vi "Record Fiducial.vi"(9 "CH index":i32, 10 "XYZ":dbl[](array[numeric]), 11 "input cluster":T1) -> (2 "All fiducials recorded":bool, 3 "output cluster":T1)   [LabVIEW 2021, in "Component Tray.lvclass"]
uses:
  Component Tray.lvclass
  Find Component.ctl
  Controller/Camera/Machine Vision.ctl
  Controller/Camera/Camera.lvclass
panel:
  out "XYZTheta":dbl[](array[numeric]) format="%.6g"
  out "CH1 XYZ":dbl[](array[numeric])
  out "Sensor ID Location":dbl[](array[numeric])
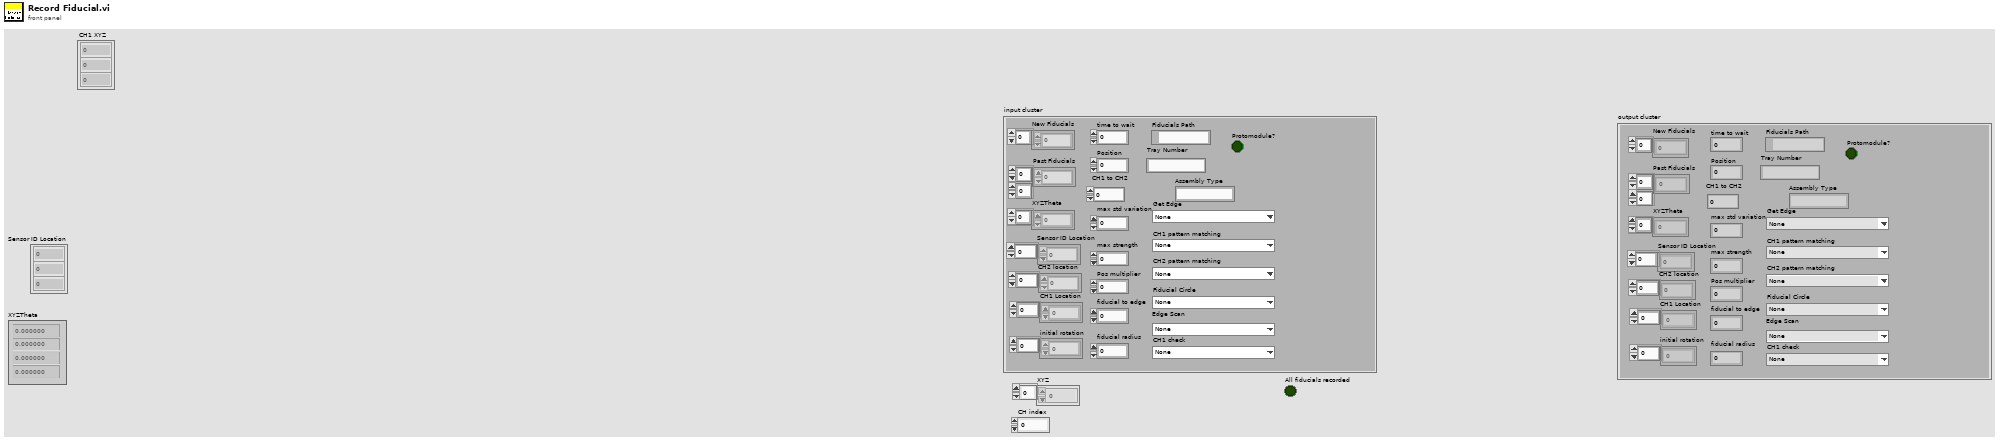
[diagram p1: front panel]
types:
  T1 = typedef "Component Tray.lvclass/Find Component.ctl" = cluster{"New Fiducials":dbl[], "Past Fiducials":dbl[][], "XYZTheta":dbl[], "Fiducials Path":path, "Position":i32, "CH1 Location":dbl[], "Sensor ID Location":dbl[], "initial rotation":dbl[], "CH2 location":dbl[], "max std variation":dbl, "max strength":dbl, "CH2 pattern matching":T2, "Fiducial Circle":T2, "Get Edge":T2, "Pos multiplier":dbl, "time to wait":u32, "fiducial to edge":dbl, "Protomodule?":bool, "Assembly Type":string, "CH1 to CH2":dbl, "Tray Number":string, "fiducial radius":dbl, "4 fiducials?":bool, "CH1 check":T2, "Edge Scan":T2, "CH1 pattern matching":T2, "Sensor Thickness":dbl}
  T2 = typedef "Camera.lvclass/Machine Vision.ctl" = enum16{"None", "Assembly Tray Circle", "Assembly Tray Fiducial", "Partial Hexaboard", "sensor edge init", "HB edge init", "sensor edge pos1", "sensor edge pos2", "HB edge pos1", "HB edge pos2", "Sensor CH1-2", "HB CH1", "HB CH2", "V3 Sensor Circle", "Hexaboard Circle", "sensor CH1 check", "HB CH1 check "}
  T3 = typedef "File Paths.ctl" = cluster{"Glue Pattern Folder":path, "Carrier Tray Folder":path, "Pick Up Tool Fixture Folder":path, "Components Folder":path, "Bellows Tool Offset.txt":path, "Pick Up Tool Offset.txt":path, "Dispense Tip Offset.txt":path, "Log Files":path, "Gantry Assembly Map.txt":path, "Syringe and offset map.txt":path, "Controllers Folder":path, "Local dbase config":path}
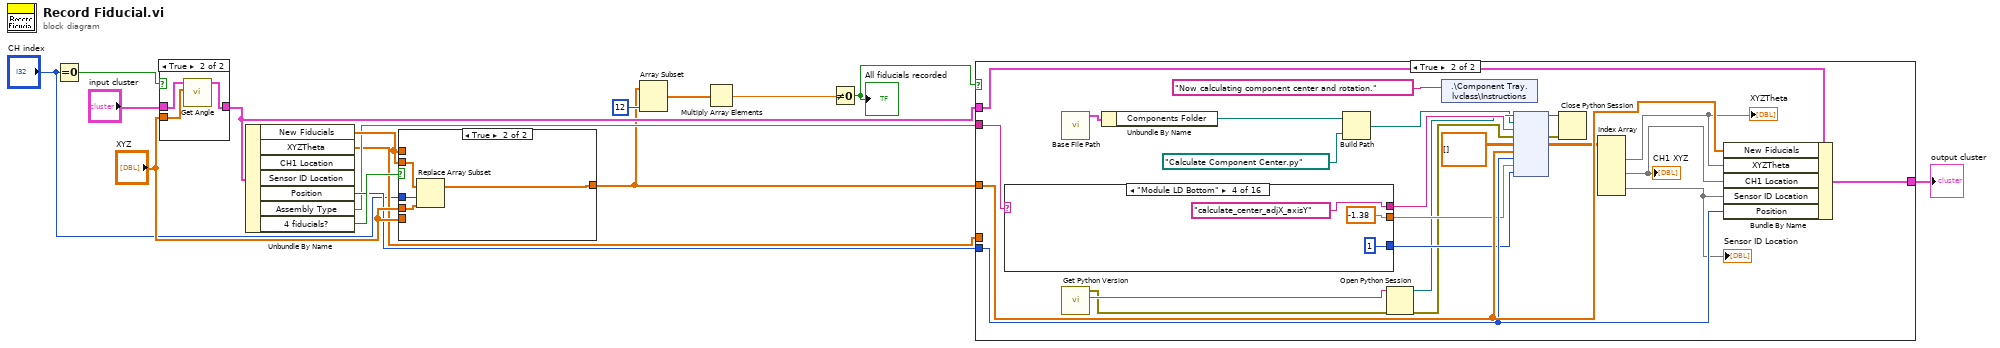
[diagram p0: block diagram]
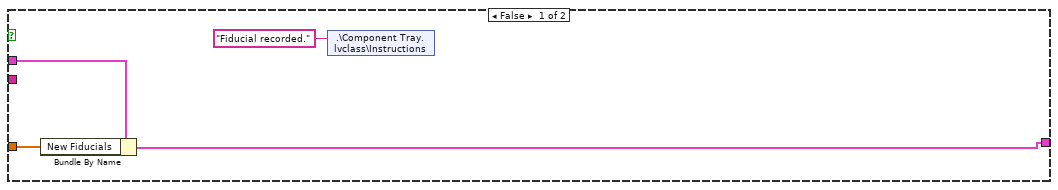
[diagram p2: hidden frame]
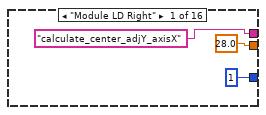
[diagram p3: hidden frame]
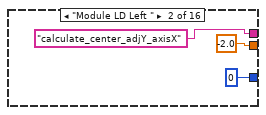
[diagram p4: hidden frame]
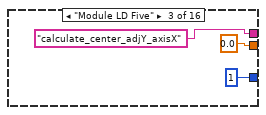
[diagram p5: hidden frame]
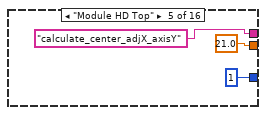
[diagram p6: hidden frame]
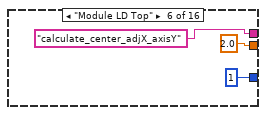
[diagram p7: hidden frame]
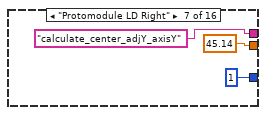
[diagram p8: hidden frame]
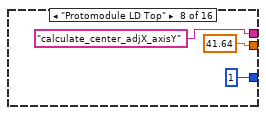
[diagram p9: hidden frame]
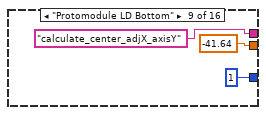
[diagram p10: hidden frame]
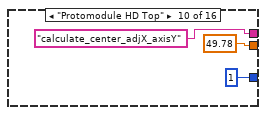
[diagram p11: hidden frame]
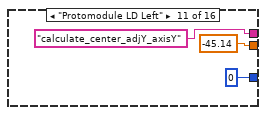
[diagram p12: hidden frame]
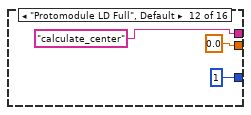
[diagram p13: hidden frame]
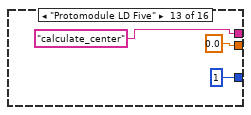
[diagram p14: hidden frame]
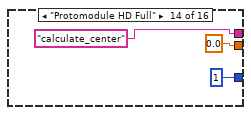
[diagram p15: hidden frame]
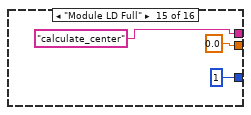
[diagram p16: hidden frame]
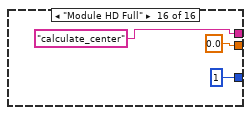
[diagram p17: hidden frame]
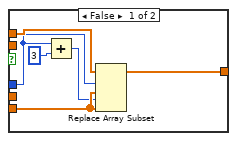
[diagram p19: hidden frame]
diagram:
  n1 = Equal To 0?(x="CH index") -> (x = 0?=w3:bool)
  n2 = case shown="True" w3 {
    tunnel: "input cluster" -> [w17 w20]
    tunnel: [w17 w19] -> w5
    tunnel: "XYZ" -> [_ w18]
    frame False {
    }
    frame True {
      n3 = call "Get Angle.vi"("array"=w18, "input cluster"=w20) -> ("output cluster"=w19:T1)  [unwired: 8 in, 1 out]
    }
  }
  n4 = Unbundle By Name(w5) -> ("New Fiducials"=w16:dbl[], "XYZTheta"=w6:dbl[], "Position"=w8:i32, "Assembly Type"=w7:string, "4 fiducials?"=w15:bool)  [unwired: 2 out]
  n5 = case shown="True" w15 {
    tunnel: w16 -> [w26 _]
    tunnel: "XYZ" -> [w25 _]
    tunnel: [w22 w27] -> w2
    tunnel: w16 -> [_ w30]
    tunnel: "XYZ" -> [_ w29]
    tunnel: "CH index" -> [w21 w28]
    frame False {
      n6 = Add(x=w21, y=3) -> (x+y=w23:i32)
      n7 = Replace Array Subset "Replace Array Subset"(array=w26, new element #1=w25, index #1=w21, new element #2=w25, index #2=w23) -> (w22:dbl[])
    }
    frame True {
      n8 = Replace Array Subset "Replace Array Subset"(array=w30, new element=w29, index=w28) -> (w27:dbl[])
    }
  }
  n9 = Array Subset "Array Subset"(array=w2, length=12) -> (w10:dbl[])  [unwired: 1 in]
  n10 = Multiply Array Elements(1:w10) -> (0:w11:dbl)
  n11 = Not Equal To 0?(x=w11) -> (x != 0?=w9:bool)
  "All fiducials recorded" <- w9
  n12 = case shown="True" w9 {
    tunnel: w2 -> [w33 w58]
    tunnel: w6 -> [_ _]
    tunnel: w8 -> [_ w57]
    tunnel: w5 -> [w34 w56]
    tunnel: [w32 w55] -> w1
    tunnel: w7 -> [_ w54]
    frame False {
      n13 = Bundle By Name(cluster=w34, "New Fiducials"=w33) -> (w32:T1)
      n14 = shared-variable ".\\Component Tray.lvclass\\Instructions"("Fiducial recorded." ("Instructions")) -> ()  [unwired: 1 in, 1 out]
    }
    frame True {
      n15 = case shown="\"Module LD Bottom\"" w54 {
        tunnel: ["calculate_center_adjY_axisX" ("function name") "calculate_center_adjY_axisX" ("function name") "calculate_center_adjY_axisX" ("function name") "calculate_center_adjX_axisY" ("function name") "calculate_center_adjX_axisY" ("function name") "calculate_center_adjX_axisY" ("function name") "calculate_center_adjY_axisY" ("function name") "calculate_center_adjX_axisY" ("function name") "calculate_center_adjX_axisY" ("function name") "calculate_center_adjX_axisY" ("function name") "calculate_center_adjY_axisY" ("function name") "calculate_center" ("function name") "calculate_center" ("function name") "calculate_center" ("function name") "calculate_center" ("function name") "calculate_center" ("function name")] -> w50
        tunnel: [28.0 -2.0 0.0 -1.38 21.0 2.0 45.14 41.64 -41.64 49.78 -45.14 0.0 0.0 0.0 0.0 0.0] -> w49
        tunnel: [1 0 1 1 1 1 1 1 1 1 0 1 1 1 1 1] -> w48
        frame "Module LD Right" {
        }
        frame "Module LD Left " {
        }
        frame "Module LD Five" {
        }
        frame "Module LD Bottom" {
        }
        frame "Module HD Top" {
        }
        frame "Module LD Top" {
        }
        frame "Protomodule LD Right" {
        }
        frame "Protomodule LD Top" {
        }
        frame "Protomodule LD Bottom" {
        }
        frame "Protomodule HD Top" {
        }
        frame "Protomodule LD Left" {
        }
        frame "Protomodule LD Full", Default {
        }
        frame "Protomodule LD Five" {
        }
        frame "Protomodule HD Full" {
        }
        frame "Module LD Full" {
        }
        frame "Module HD Full" {
        }
      }
      n16 = call "Base File Path.vi"() -> ("Paths Out"=w43:T3)  [unwired: 11 in]
      n17 = call "Get Python Version.vi"() -> ("Python Version"=w37:string, "error out"=w36:errorcluster)  [unwired: 10 in]
      n18 = Unbundle By Name(w43) -> ("Components Folder"=w41:path)
      n19 = Build Path(base path=w41, name or relative path=path "Calculate Component Center.py") -> (appended path=w40:path)
      n20 = Open Python Session(python version=w37, 3:w36) -> (session out=w47:refnum<k35>, error out=w45:errorcluster)  [unwired: 1 in]
      n21 = shared-variable ".\\Component Tray.lvclass\\Instructions"("Now calculating component center and rotation." ("Instructions")) -> ()  [unwired: 1 in, 1 out]
      n22 = node(w47, w40, w50, w45, dbl[][] [], w58, w57, w49, w48) -> (w46:refnum<k35>, w44:errorcluster, w38:dbl[][])  [unwired: 4 in, 2 out]
      n23 = Close Python Session(session in=w46, error in=w44) -> ()  [unwired: 1 out]
      n24 = Index Array(array=w38) -> (element #1=w51:dbl[], element #2=w52:dbl[], element #3=w53:dbl[])  [unwired: 6 in]
      "XYZTheta" <- w51
      "CH1 XYZ" <- w52
      "Sensor ID Location" <- w53
      n25 = Bundle By Name(cluster=w56, "New Fiducials"=w58, "XYZTheta"=w51, "CH1 Location"=w52, "Sensor ID Location"=w53, "Position"=w57) -> (w55:T1)
    }
  }
  "output cluster" <- w1
